vi "setWindow.vi"(8 "Error In":errorcluster, 10 "window":refnum<class "QWindow.lvclass">, 11 "QWinTaskbarButton In":refnum<class "QWinTaskbarButton.lvclass">) -> (0 "Error Out":errorcluster, 3 "QWinTaskbarButton Out":refnum<class "QWinTaskbarButton.lvclass">)   [LabVIEW 2014, in "QWinTaskbarButton.lvclass"]
doc: "LabVIEW-specific documentation is not yet available. See <b>https://doc.qt.io/qt-5/qwintaskbarbutton.html#setWindow</b>"
uses:
  QWinTaskbarButton.lvclass
  Qt GUI/QWindow/QWindow.lvclass
  LQ Core/LQIdentity/LQIdentity.lvclass/LQIdentity.ctl
  LQ Core/LQ Core.lvlib
  LQ Core/LQIdentity/LQIdentity.lvclass
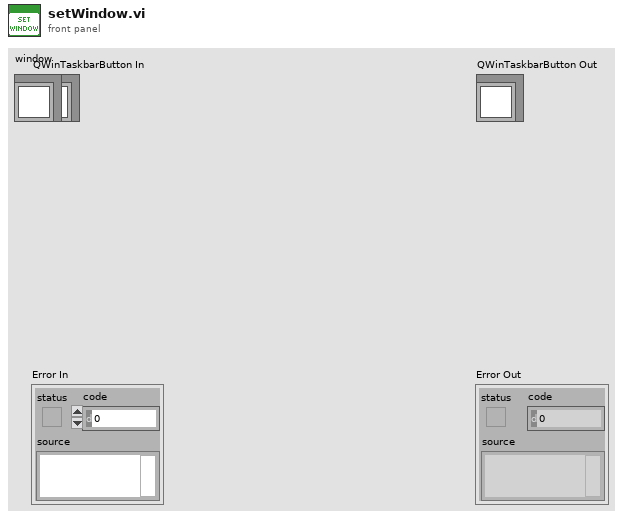
[diagram p1: front panel]
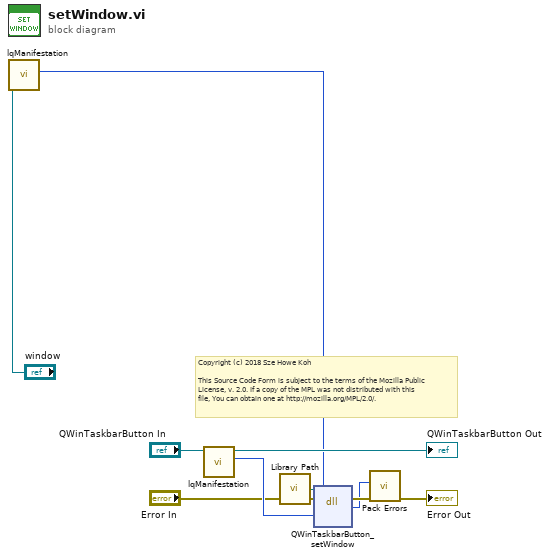
[diagram p0: block diagram]
diagram:
  # "Copyright (c) 2018 Sze Howe Koh\n\nThis Source Code Form is subject to the terms of the Mozilla Public\nLicense, v. 2.0. If a copy of the MPL was not distributed with this\nfile, You can obtain one at http://mozilla.org/MPL/2.0/."
  n1 = call "lqManifestation.vi"("LQIdentity in"="window") -> ("Manifestation"=w1:u64)  [unwired: 9 in, 1 out]
  n2 = call "lqManifestation.vi"("LQIdentity in"="QWinTaskbarButton In") -> ("Manifestation"=w7:u64, "LQIdentity out"=→"QWinTaskbarButton Out":refnum<class "QWinTaskbarButton.lvclass">)  [unwired: 9 in]
  n3 = call "Library Path.vi"() -> ("Library Path"=w8:path)
  n4 = dll-call lib="?" fn="QWinTaskbarButton_setWindow"(path in=w8, error in="Error In", "_instance"=w7, "window"=w1) -> (error out=w5:errorcluster, w3:i32)  [unwired: 3 in, 1 out]
  n5 = call "Pack Errors.vi"("Error In"=w5, "Error Code"=w3) -> ("Error Out"=→"Error Out":errorcluster)  [unwired: 9 in]
